vi "Add BrowerTree Component.vi"(6 "SymbolIndex":T1, 8 "error in (no error)":errorcluster, 9 "Left Cell String":string, 10 "Parent Tag":string, 11 "BrowerTree in":refnum<class "BrowerTree.lvclass">) -> (0 "error out":errorcluster, 2 "BrowerComponentID(\"\")":string, 3 "BrowerTree out":refnum<class "BrowerTree.lvclass">)   [LabVIEW 2015, in "BrowerTree.lvclass"]
uses:
  BrowerTree.lvclass
  Type Definition/Symbol Index.ctl
  BrowerTree.lvclass/BrowerTree.ctl
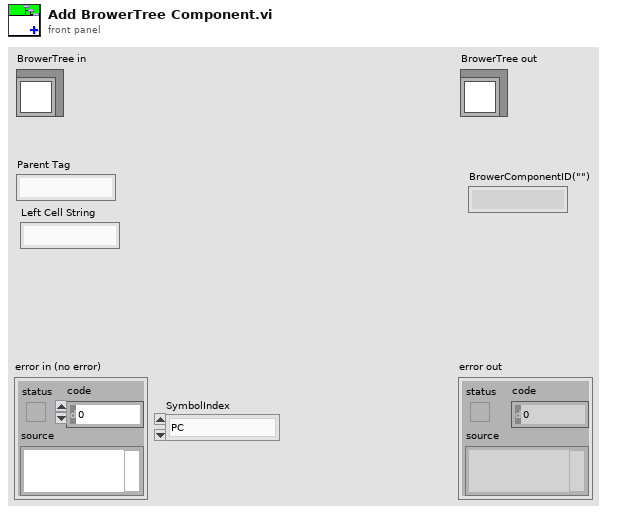
[diagram p1: front panel]
types:
  T1 = typedef "BrowerTree.lvclass/Symbol Index.ctl" = enum16{"PC", "Project", "Module", "DebugTask", "Communication"}
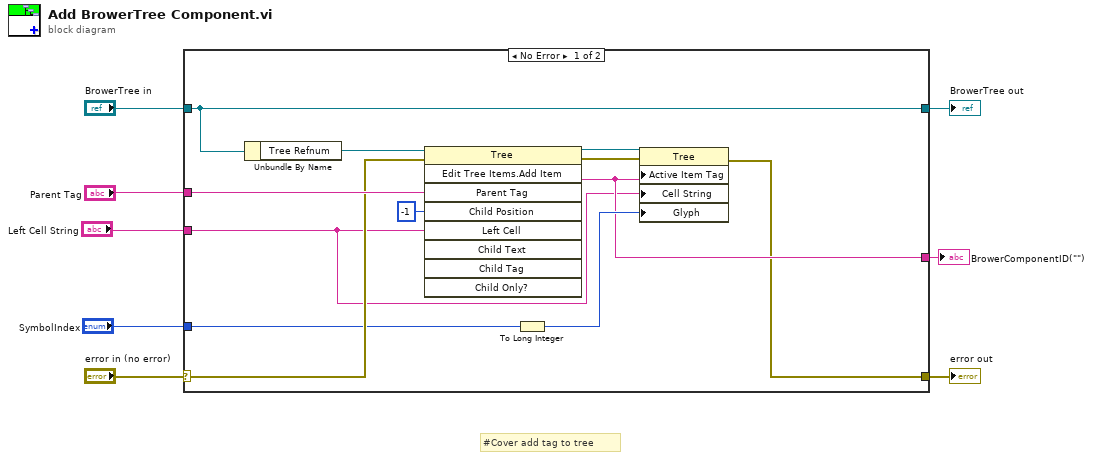
[diagram p0: block diagram]
diagram:
  # "#Cover add tag to tree"
  n1 = case shown="No Error" "error in (no error)" {
    selector: "error in (no error)" -> [w14 w22]
    tunnel: [w10 w22] -> w7
    tunnel: [w20 w21] -> w5
    tunnel: "BrowerTree in" -> [w20 w21]
    tunnel: "Parent Tag" -> [w18 _]
    tunnel: "SymbolIndex" -> [w13 _]
    tunnel: [w11 _] -> w2
    tunnel: "Left Cell String" -> [w9 _]
    frame No Error {
      n2 = Unbundle By Name(w20) -> ("Tree Refnum"=w19:refnum<vi>)
      n3 = invoke class="Tree" method="Edit Tree Items.Add Item"(reference=w19, error in=w14, "Parent Tag"=w18, "Child Position"=-1, "Left Cell"=w9) -> (reference out=w16:refnum<vi>, error out=w15:errorcluster, "Edit Tree Items:Add Item"=w11:string)  [unwired: 4 in, 6 out]
      n4 = To Long Integer(number=w13) -> (32bit integer=w12:i32)
      n5 = property class="Tree"(reference=w16, error in=w15, "Active Item Tag"=w11, "Cell String"=w9, "Glyph"=w12) -> (error out=w10:errorcluster)  [unwired: 1 out]
    }
    frame Error {
    }
  }
  "error out" <- w7
  "BrowerTree out" <- w5
  "BrowerComponentID(\"\")" <- w2
